vi "Configure Measurement (Voltage).vi"(0 "VISA resource name":refnum<visa-resource-name>, 1 "Channel (0: Channel 1)":i32(ring) items=["Channel 1", "Channel 2"], 3 "Voltage Range (2 V)":dbl=2.0, 5 "error in (no error)":errorcluster, 6 "Auto Voltage NPLC(F: Disable)":bool, 7 "Voltage NPLC (0.1 PLC)":dbl=0.1, 10 "Voltage Auto Range (T: Enable)":bool=TRUE, 11 "Voltage Range Lower Limit (0.2 V)":dbl=0.2, 12 "Voltage Auto Range Mode (0: Normal)":i32(ring) items=["Normal", "Resolution", "Speed"], 13 "Voltage Auto Range Threshold Rate (50 percent)":dbl=50.0) -> (14 "VISA resource name out":refnum<visa-resource-name>, 19 "error out":errorcluster)   [LabVIEW 2026, in "Agilent B2900 Series.lvlib"]
doc: "Configures the settings for voltage measurement function.\n\n<B>Note:</B>\nCommands in default part of the case structure are not applicable for Agilent models B2961A, B2962A, B2961B,B2962B,B2961C and B2962C."
uses:
  Agilent B2900 Series.lvlib
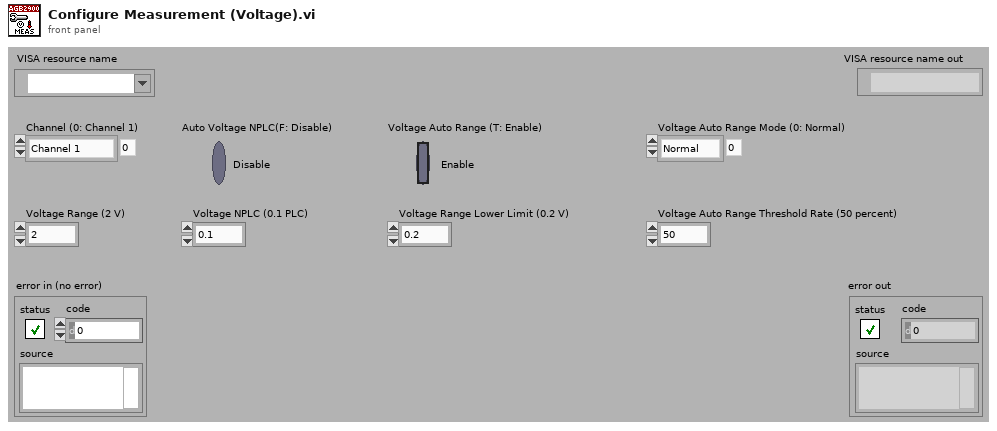
[diagram p1: front panel]
types:
  T1 = typedef "Agilent B2900 Series.lvlib/Extended User Data.ctl" = cluster{"B2900 Series Mode":u16}
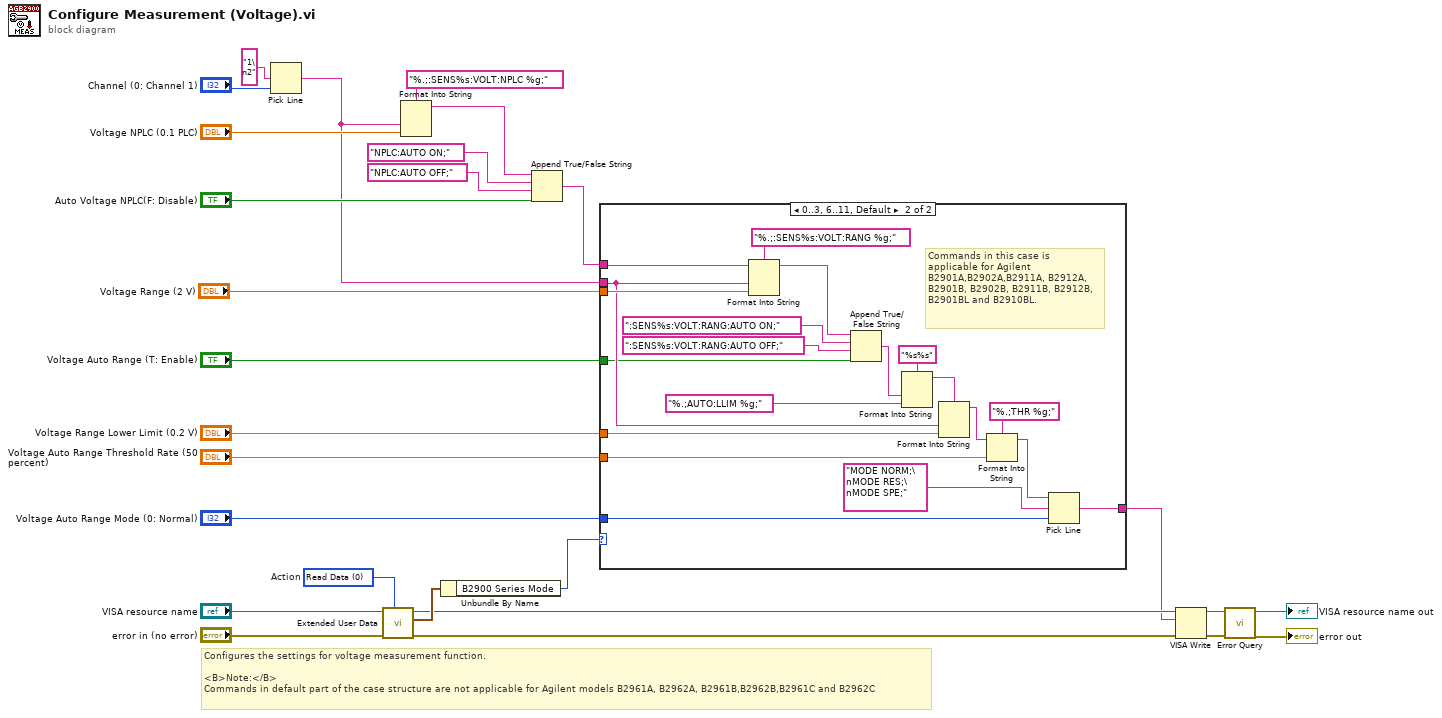
[diagram p0: block diagram]
diagram:
  w16 = 0 items=["Read Data", "Write Data", "Clear Data", "Clear ALL Data"]  # Action
  # "Configures the settings for voltage measurement function.\n\n<B>Note:</B>\nCommands in default part of the case structure are not applicable for Agilent models B2961A, B2962A, B2961B,B2962B,B2961C and B2962C"
  n1 = Pick Line(multi-line string="1\n2" ("string (\"\")"), line index="Channel (0: Channel 1)") -> (output string=w8:string)  [unwired: 1 in]
  n2 = call "Extended User Data.vi"("Action (1: Write Data)"=w16, "Error In (no error)"="error in (no error)", "VISA resource name in"="VISA resource name") -> ("Error Out"=w11:errorcluster, "User Data Out"=w15:T1, "VISA resource name out"=w12:refnum<visa-resource-name>)  [unwired: 6 in]
  n3 = Format Into String(format string="%.;:SENS%s:VOLT:NPLC %g;", w8, "Voltage NPLC (0.1 PLC)") -> (resulting string=w10:string)  [unwired: 2 in, 1 out]
  n4 = Unbundle By Name(w15) -> ("B2900 Series Mode"=w3:u16)
  n5 = Append True/False String(1:"Auto Voltage NPLC(F: Disable)", 2:"NPLC:AUTO OFF;", 3:"NPLC:AUTO ON;", 4:w10) -> (0:w1:string)
  n6 = case shown="0..3, 6..11, Default" w3 {
    tunnel: "Voltage Range (2 V)" -> [_ w36]
    tunnel: w8 -> [_ w35]
    tunnel: "Voltage Auto Range (T: Enable)" -> [_ w34]
    tunnel: "Voltage Range Lower Limit (0.2 V)" -> [_ w33]
    tunnel: "Voltage Auto Range Threshold Rate (50 percent)" -> [_ w32]
    tunnel: "Voltage Auto Range Mode (0: Normal)" -> [_ w31]
    tunnel: [w28 w30] -> w2
    tunnel: w1 -> [w28 w29]
    frame 4, 5, 12, 13 {
      # "Commands in this case are\napplicable for Agilent B2961A,B2962A, B2961B, B2962B."
    }
    frame 0..3, 6..11, Default {
      # "Commands in this case is applicable for Agilent B2901A,B2902A,B2911A, B2912A, B2901B, B2902B, B2911B, B2912B, B2901BL and B2910BL."
      n7 = Format Into String(format string="%.;:SENS%s:VOLT:RANG %g;", initial string=w29, w35, w36) -> (resulting string=w48:string)  [unwired: 1 in, 1 out]
      n8 = Append True/False String(1:w34, 2:":SENS%s:VOLT:RANG:AUTO OFF;", 3:":SENS%s:VOLT:RANG:AUTO ON;", 4:w48) -> (0:w45:string)
      n9 = Format Into String(format string="%s%s", w45, "%.;AUTO:LLIM %g;") -> (resulting string=w47:string)  [unwired: 2 in, 1 out]
      n10 = Format Into String(format string=w47, w35, w33) -> (resulting string=w40:string)  [unwired: 2 in, 1 out]
      n11 = Format Into String(format string="%.;THR %g;", initial string=w40, w32) -> (resulting string=w43:string)  [unwired: 1 in, 1 out]
      n12 = Pick Line(string ("")=w43, multi-line string="MODE NORM;\nMODE RES;\nMODE SPE;", line index=w31) -> (output string=w30:string)
    }
  }
  n13 = VISA Write(VISA resource name=w12, write buffer=w2, error in (no error)=w11) -> (VISA resource name out=w22:refnum<visa-resource-name>, error out=w21:errorcluster)  [unwired: 1 out]
  n14 = call "Error Query.vi"("error in (no error)"=w21, "VISA resource name"=w22) -> ("error out"=→"error out":errorcluster, "VISA resource name out"=→"VISA resource name out":refnum<visa-resource-name>)  [unwired: 6 in, 2 out]
